vi "random_bytes.vi"(11 "length (18bytes)":i32=18) -> (3 "random bytes":string)   [LabVIEW 2022 SP3, in "LabVIEW-Hashlib.lvlib"]
doc: "Generates random bytes.\n\nCreated by: Ryan Pacini"
uses:
  LabVIEW-Hashlib.lvlib
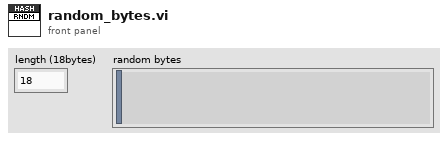
[diagram p1: front panel]
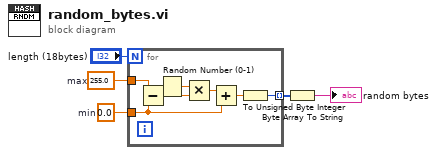
[diagram p0: block diagram]
diagram:
  w3 = 0.0  # min
  w4 = 255.0  # max
  n1 = for {
    N: "length (18bytes)" -> [_]
    tunnel: [w8] -> w2 mode=indexing
    tunnel: w4 -> [w7]
    tunnel: w3 -> [w6]
    n2 = Subtract(x=w7, y=w6) -> (x-y=w11:dbl)
    n3 = Random Number (0-1)() -> (number: 0 to 1=w12:dbl)
    n4 = Multiply(x=w12, y=w11) -> (x*y=w10:dbl)
    n5 = Add(x=w10, y=w6) -> (x+y=w9:dbl)
    n6 = To Unsigned Byte Integer(number=w9) -> (unsigned 8bit integer=w8:u8)
  }
  n7 = Byte Array To String(unsigned byte array=w2) -> (string=→"random bytes":string)
